vi "Pause.vi"(8 "error in (no error)":errorcluster, 11 "Sequence in":refnum<class "Sequence.lvclass">) -> (0 "error out":errorcluster, 1 "SeqPaused":bool, 3 "Sequence out":refnum<class "Sequence.lvclass">)   [LabVIEW 2019, in "Sequence.lvclass"]
uses:
  Sequence.lvclass
  Sequence.lvclass/Sequence.ctl
  Datalog/DatalogSubvis/SearchableTag.ctl
  SequenceSubvis/RF Direction.ctl
  SequenceSubvis/PolarizationSelect.ctl
  Support/MessageAPI/UIMessage.ctl
  SendMessage/SendMessage.lvclass
  Datalog/DataLog.lvclass
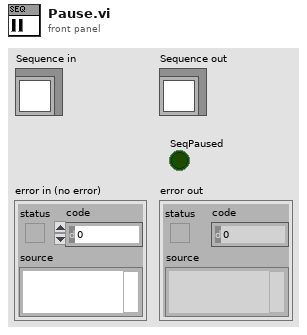
[diagram p1: front panel]
types:
  T1 = typedef "UIMessage.ctl" = cluster{"EventCode":i32, "Numeric":dbl, "String":string, "Variant":variant}
  T2 = typedef "DataLog.lvclass/SearchableTag.ctl" = cluster{"Module, 0-63":i32, "RF Direction Tx0":T3, "Polarization, V0 H1":T4, "AO-64 Array":dbl[]}
  T3 = typedef "RF Direction.ctl" = enum16{"Tx - RF In", "Rx - RF Out"}
  T4 = typedef "PolarizationSelect.ctl" = enum16{"Vertical", "Horizontal"}
  T5 = typedef "mWaveTestStep.ctl" = cluster{"StepType":T6, "RF In/Out":T3, "Module/Raster":i32, "Polarization":T4, "AO-64 Array":dbl[], "Position":T7[]}
  T6 = typedef "TestStepTypes.ctl" = enum16{"MotionFF-M2", "Motion", "SweepTest", "RasterTest", "Finish", "64ModuleCfg"}
  T7 = typedef "singleAxisMoveDef.ctl" = cluster{"mmWave Axis":T8, "eng. value":dbl}
  T8 = typedef "mmWaveAxis.ctl" = string
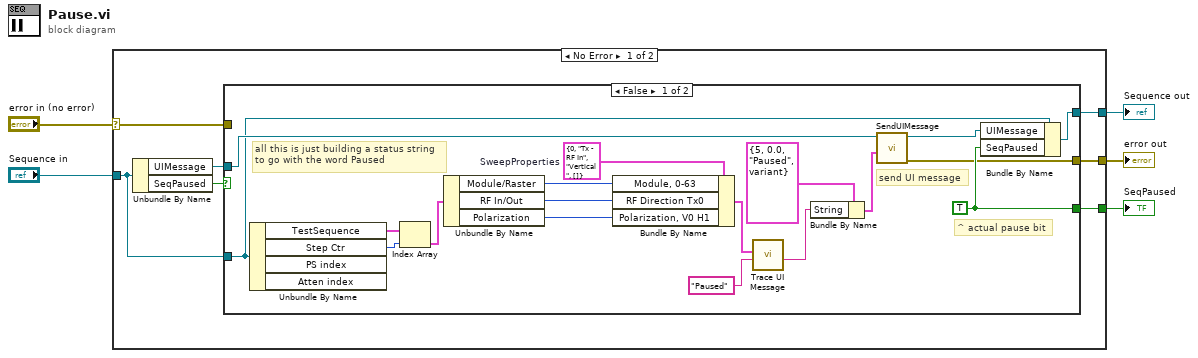
[diagram p0: block diagram]
diagram:
  n1 = case shown="No Error" "error in (no error)" {
    selector: "error in (no error)" -> [w6 w34]
    tunnel: [w7 w34] -> w4
    tunnel: [w9 w33] -> w3
    tunnel: "Sequence in" -> [w10 w33]
    tunnel: [w11 _] -> w2
    frame No Error {
      n2 = Unbundle By Name(w10) -> ("UIMessage"=w8:refnum<class "SendMessage.lvclass">, "SeqPaused"=w12:bool)
      n3 = case shown="False" w12 {
        tunnel: [w29 _] -> w11
        tunnel: [w30 w32] -> w9
        tunnel: w10 -> [w14 w32]
        tunnel: w8 -> [w28 _]
        tunnel: [w26 w31] -> w7
        tunnel: w6 -> [_ w31]
        frame False {
          w21 = T2 {"Module, 0-63"=0, "RF Direction Tx0"=enum."Tx - RF In", "Polarization, V0 H1"=enum."Vertical", "AO-64 Array"=[]}  # SweepProperties
          w29 = TRUE
          # "^ actual pause bit"
          # "all this is just building a status string\nto go with the word Paused"
          # "send UI message"
          n4 = Unbundle By Name(w14) -> ("TestSequence"=w25:T5[], "Step Ctr"=w24:i32)  [unwired: 2 out]
          n5 = Index Array(array=w25, index=w24) -> (element=w23:T5)
          n6 = Unbundle By Name(w23) -> ("Module/Raster"=w20:i32, "RF In/Out"=w19:T3, "Polarization"=w18:T4)
          n7 = Bundle By Name(cluster=w21, "Module, 0-63"=w20, "RF Direction Tx0"=w19, "Polarization, V0 H1"=w18) -> (w16:T2)
          n8 = call "Trace UI Message.vi"("Command"="Paused" ("String"), "SweepProperties"=w16) -> ("UI Msg String"=w15:string)  [unwired: 9 in]
          n9 = Bundle By Name(cluster=T1 {"EventCode"=5, "Numeric"=0.0, "String"="Paused", "Variant"=variant} ("UIMsg"), "String"=w15) -> (w13:T1)
          n10 = call-dynamic "SendUIMessage.vi"("UIMsg"=w13, "SendMessage in"=w28) -> ("error out"=w26:errorcluster, "SendMessage out"=w27:refnum<class "SendMessage.lvclass">)  [unwired: 8 in]
          n11 = Bundle By Name(cluster=w14, "UIMessage"=w27, "SeqPaused"=w29) -> (w30:refnum<class "Sequence.lvclass">)
        }
        frame True {
        }
      }
    }
    frame Error {
    }
  }
  "error out" <- w4
  "Sequence out" <- w3
  "SeqPaused" <- w2
